vi "Is Owner Null.vi"(8 "error in (no error)":errorcluster, 11 "Config Element in":refnum<class "Config Element.lvclass">) -> (0 "error out":errorcluster, 2 "Owner Null":bool, 3 "Config Element out":refnum<class "Config Element.lvclass">)   [LabVIEW 2020, in "CDM-Config.lvlib" / "Config Element.lvclass"]
uses:
  Config Element.lvclass
  Config Element.lvclass/Config Element.ctl
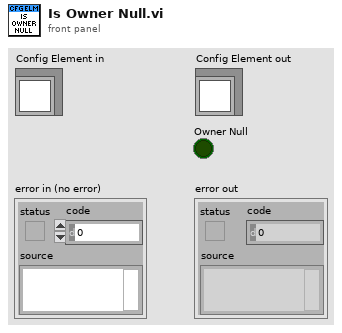
[diagram p1: front panel]
types:
  T1 = typedef "CDM-Config.lvlib/Config Element.lvclass/Ref Data.ctl" = cluster{"Node Info":T2, "Owner":refnum<class>, "Changed":bool, "Name":string, "Value":string, "Meta Data":T3[]}
  T2 = typedef "CDM-Config.lvlib/Node Info.ctl" = cluster{"Index":i32, "Parent":i32, "Children":i32[]}
  T3 = typedef "CDM-Config.lvlib/Meta Data.ctl" = cluster{"Name":string, "Value":string}
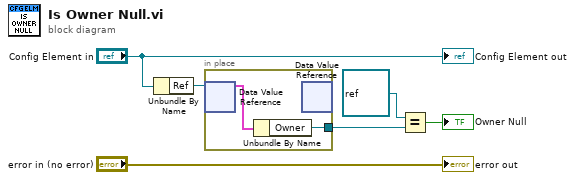
[diagram p0: block diagram]
diagram:
  n1 = Unbundle By Name("Config Element in") -> ("Ref"=w5:refnum<data-value>)
  n2 = in-place {
    in-place-border: [w7] -> w3
    n3 = in-place-dvr #1(w5) -> (w8:T1)  [unwired: 1 out]
    n4 = Unbundle By Name(w8) -> ("Owner"=w7:refnum<class>)
    n5 = in-place-dvr #1() -> ()  [unwired: 1 in, 2 out]
  }
  n6 = Equal?(x=refnum<class> refnum, y=w3) -> (x = y?=→"Owner Null":bool)
  "error out" <- "error in (no error)"
  "Config Element out" <- "Config Element in"
